vi "dialog box.vi"(4 "State":i16, 5 "Time":dbl format="%.2f", 6 "Sensor Values":dbl[](array[numeric]), 7 "Set Points":dbl[](array[numeric])) -> (0 "required data":T1={"Set Point names"=["state to reset counter", "state to count"], "required number of setpoints"=2, "required number of sensors"=0, "Sensor names"=[]}, 3 "output value":dbl)   [LabVIEW 2019]
panel:
  # "Enter the correct information for this control code in the required data structure below. Then make the current value default by right clicking on the border of the data structure. Select \"data operations\" and then select \"make current value default\". These values will be displayed by process controller."
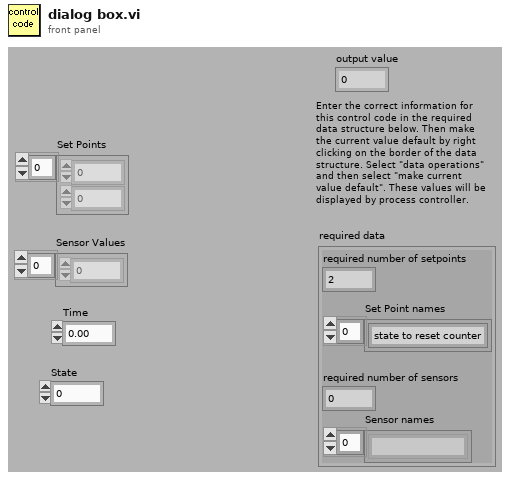
[diagram p1: front panel]
types:
  T1 = cluster{"Set Point names":string[], "required number of setpoints":u8, "required number of sensors":u8, "Sensor names":string[]}
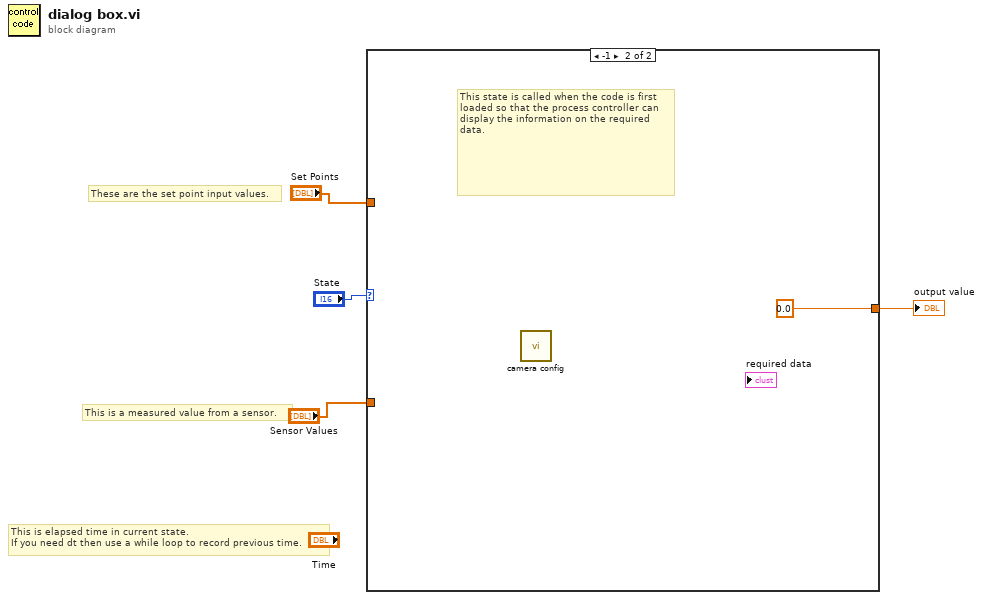
[diagram p0: block diagram]
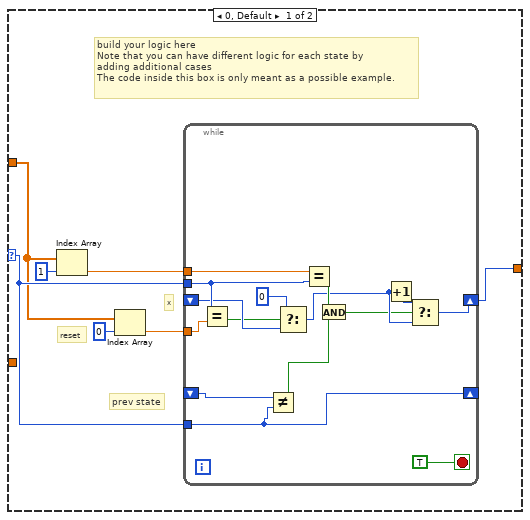
[diagram p2: hidden frame]
diagram:
  # "These are the set point input values."
  # "This is a measured value from a sensor."
  # "This is elapsed time in current state.\nIf you need dt then use a while loop to record previous time."
  n1 = case shown="-1" "State" {
    selector: "State" -> [w9 _]
    tunnel: [w5 0.0 ("fraction on")] -> w3
    tunnel: "Set Points" -> [w6 _]
    tunnel: "Sensor Values" -> [_ _]
    frame 0, Default {
      # "prev state"
      # "reset"
      # "x"
      # "build your logic here\nNote that you can have different logic for each state by\nadding additional cases\nThe code inside this box is only meant as a possible example."
      n2 = Index Array(array=w6, index=1) -> (element=w10:dbl)
      n3 = Index Array(array=w6, index=0) -> (element=w7:dbl)
      n4 = while {
        shift-right: [w25] -> _
        shift-left: _ -> [w16]
        tunnel: w9 -> [w25]
        tunnel: w10 -> [w26]
        tunnel: w9 -> [w19]
        shift-right: [w23] -> w5
        shift-left: _ -> [w15]
        tunnel: w7 -> [w18]
        stop <- TRUE stop-if-true
        n5 = Equal?(x=w19, y=w18) -> (x = y?=w13:bool)
        n6 = Not Equal?(x=w16, y=w25) -> (x != y?=w24:bool)
        n7 = Select(t=0, s=w13, f=w15) -> (s? t:f=w17:i32)
        n8 = Equal?(x=w26, y=w19) -> (x = y?=w21:bool)
        n9 = And(x=w21, y=w24) -> (x .and. y?=w12:bool)
        n10 = Increment(x=w17) -> (x+1=w20:i32)
        n11 = Select(t=w20, s=w12, f=w17) -> (s? t:f=w23:i32)
      }
    }
    frame -1 {
      # "This state is called when the code is first loaded so that the process controller can display the information on the required data."
      n12 = call "camera config.vi"() -> ()  [unwired: 12 in]
    }
  }
  "output value" <- w3
